vi "HandleCmd.vi"(8 "error in (no error)":errorcluster, 11 "PM_Group in":refnum<class "PM_Group.lvclass">) -> (0 "error out":errorcluster, 3 "PM_Group out":refnum<class "PM_Group.lvclass">)   [LabVIEW 2019, in "PM_Group.lvclass"]
uses:
  PM_Group.lvclass
  D:/GIT H4000/H4000/src/Device_class/Device.lvclass
  Device_class/Device.lvclass/Device.ctl
  Proccess_class/Proccess.lvclass/Proccess.ctl
  TypeDef/GUI Setting PMG.ctl
  PM_Group.lvclass/PM_Group.ctl
  SV_Puplisher_class/SV_Publisher.lvclass/SV_Publisher.ctl
  TypeDef/Active Motor.ctl
  TypeDef/Motor N.ctl
  0e91dc30-495c-4c1b-9970-a125a349d0cc.vi
  4c1e5f9d-d6a2-473c-8de3-15165af54c15.vi
  Proccess_class/GetNames.vi
  Proccess_class/GetLogger.vi
  SV_Puplisher_class/Set SV.vi/1ae5d02c-efd0-450a-8aa4-8388e25d05bc.vi
  Device_class/Device.lvclass
  D:/GIT H4000/H4000/src/Proccess_class/Proccess.lvclass
  Logger_class/WriteEvent.vi
  <vilib>/addons/_JKI.lib/Serialization/JSON/Library/Unflatten From JSON String.vi
  MessageInterface_class/MessageInterface.lvclass
  ConfigInterface_class/ConfigInterface.lvclass
  SV_Puplisher_class/SV_Publisher.lvclass
panel:
  out "String":string
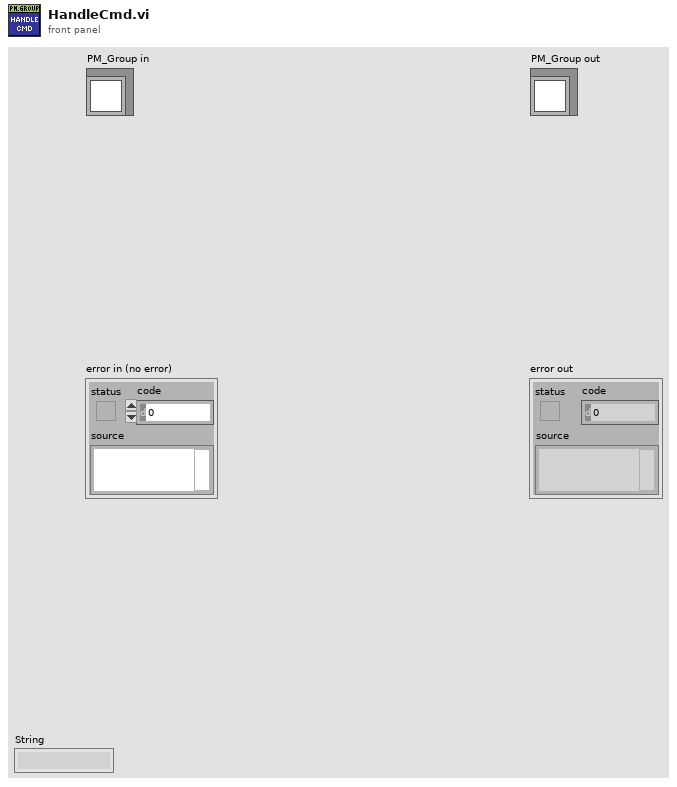
[diagram p1: front panel]
types:
  T1 = typedef "MessageInterface.lvclass/Message.ctl" = cluster{"name":string, "value":string, "receiver host":string, "receiver process":string, "source host":string, "source process":string}
  T2 = typedef "GUI Setting PMG.ctl" = cluster{"Temp Turn ON M24":dbl, "Temp Turn OFF M24":dbl, "Temp Open Water M21":dbl, "Temp Close Water M21":dbl, "H_51_on (cool)":dbl, "L_51_off (cool)":dbl, "H_52_off (oil)":dbl, "L_52_on (oil)":dbl, "filling oil delta level":dbl, "filling oil timout":dbl}
  T3 = typedef "Active Motor.ctl" = cluster{"Active":bool, "MotorN":T4}
  T4 = typedef "Motor N.ctl" = enum16{"M12", "M21", "M24"}
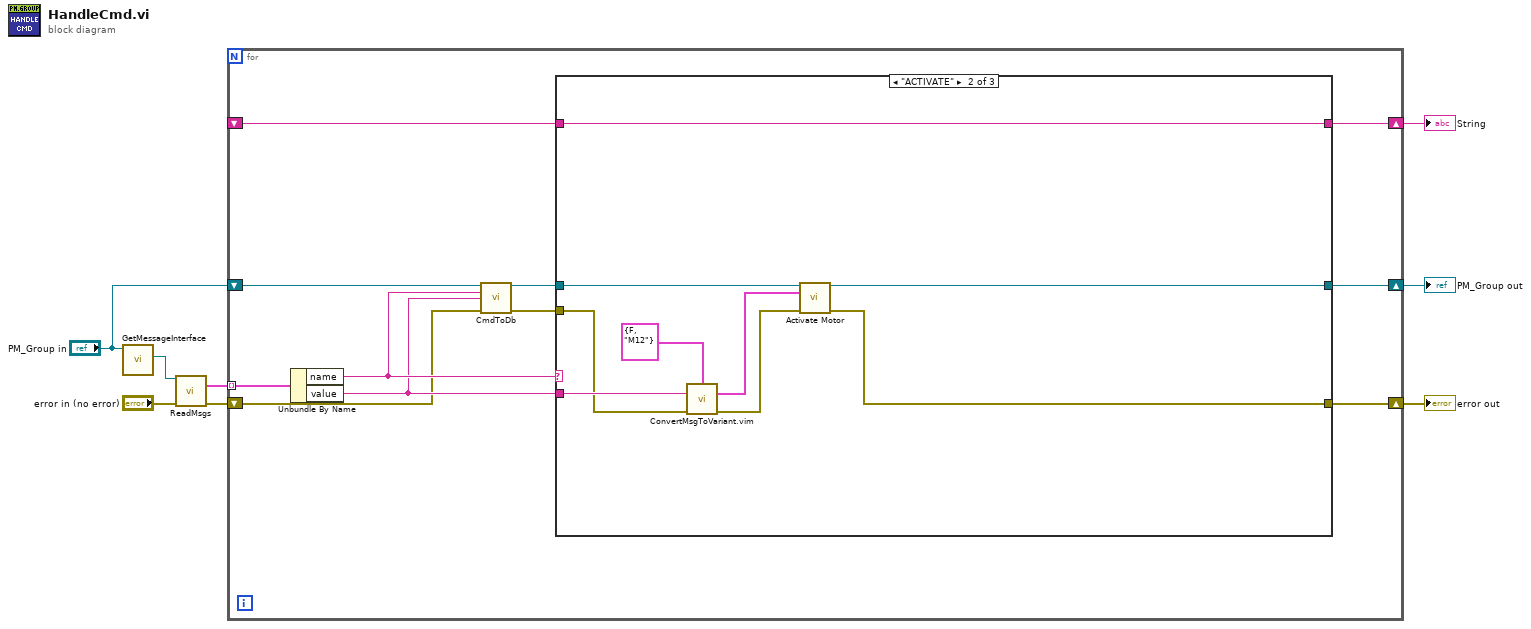
[diagram p0: block diagram]
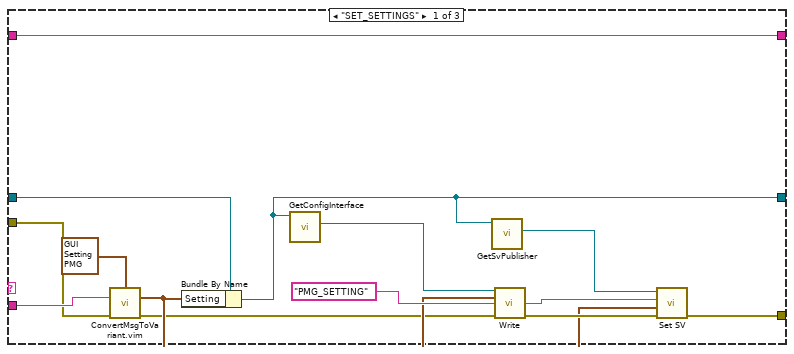
[diagram p2: hidden frame]
diagram:
  n1 = call "GetMessageInterface.vi"("Device in"="PM_Group in") -> ("MessageInterface"=w8:refnum<class "MessageInterface.lvclass">)  [unwired: 10 in]
  n2 = call-dynamic "ReadMsgs.vi"("reference in"=w8, "error in (no error)"="error in (no error)") -> ("msgs"=w6:T1[], "error out"=w7:errorcluster)  [unwired: 11 in, 1 out]
  n3 = for {
    shift-right: [w18] -> w1
    shift-left: w7 -> [w10]
    tunnel: w6 -> [w17] mode=indexing
    shift-right: [w19] -> w2
    shift-left: "PM_Group in" -> [w14]
    shift-right: [w16] -> w5
    shift-left: _ -> [w15]
    n4 = Unbundle By Name(w17) -> ("name"=w13:string, "value"=w12:string)
    n5 = call "CmdToDb.vi"("reference in"=w14, "CMD"=w13, "Value"=w12, "error in (no error)"=w10) -> ("reference out"=w11:refnum<class "PM_Group.lvclass">, "error out"=w9:errorcluster)  [unwired: 10 in]
    n6 = case shown="\"ACTIVATE\"" w13 {
      selector: w13 -> [_ _ w43]
      tunnel: [w20 w41 w45] -> w19
      tunnel: w11 -> [w29 w40 w45]
      tunnel: w9 -> [w31 w35 w44]
      tunnel: [w23 w39 w44] -> w18
      tunnel: w12 -> [w32 w38 _]
      tunnel: [w33 w42 w43] -> w16
      tunnel: w15 -> [w33 w42 _]
      frame "SET_SETTINGS" {
        n7 = call "ConvertMsgToVariant.vim"("Type and Defaults"=T2 {"Temp Turn ON M24"=0.0, "Temp Turn OFF M24"=0.0, "Temp Open Water M21"=0.0, "Temp Close Water M21"=0.0, "H_51_on (cool)"=0.0, "L_51_off (cool)"=0.0, "H_52_off (oil)"=0.0, "L_52_on (oil)"=0.0, "filling oil delta level"=0.0, "filling oil timout"=0.0} ("PMG_SETTING"), "Value"=w32, "error in (no error)"=w31) -> ("data"=w24:T2, "error out"=w21:errorcluster)  [unwired: 11 in]
        n8 = Bundle By Name(cluster=w29, "Setting"=w24) -> (w20:refnum<class "PM_Group.lvclass">)
        n9 = call "GetConfigInterface.vi"("Device in"=w20) -> ("ConfigInterface"=w28:refnum<class "ConfigInterface.lvclass">)  [unwired: 10 in]
        n10 = call "GetSvPublisher.vi"("Device in"=w20) -> ("SV_Publisher.lvclass"=w27:refnum<class "SV_Publisher.lvclass">)  [unwired: 10 in]
        n11 = call-dynamic "Write.vi"("reference in"=w28, "Data"=w24, "Name"="PMG_SETTING", "error in (no error)"=w21) -> ("Name dub"=w22:string, "error out"=w25:errorcluster)  [unwired: 8 in, 2 out]
        n12 = call "Set SV.vi"("error in (no error)"=w25, "SV Value"=w24, "SV Name"=w22, "SV_Publisher in"=w27) -> ("error out"=w23:errorcluster)  [unwired: 6 in, 1 out]
      }
      frame "ACTIVATE" {
        n13 = call "ConvertMsgToVariant.vim"("Type and Defaults"=T3 {"Active"=FALSE, "MotorN"=enum."M12"} ("Active Motor"), "Value"=w38, "error in (no error)"=w35) -> ("data"=w36:T3, "error out"=w34:errorcluster)  [unwired: 11 in]
        n14 = call "Activate Motor.vi"("reference in"=w40, "Active Motor"=w36, "error in (no error)"=w34) -> ("reference out"=w41:refnum<class "PM_Group.lvclass">, "error out"=w39:errorcluster)  [unwired: 11 in]
      }
      frame Default {
      }
    }
  }
  "error out" <- w1
  "PM_Group out" <- w2
  "String" <- w5
